vi "Average RGB Sub VI.vi"(5 "Coordinates of Overlay":cluster{"x-coord":i32, "y-coord":i32}, 7 "Transparency Factor":sgl, 8 "error in":errorcluster, 9 "Image":u32[][](array[numeric]), 10 "Overlay":u32[][](array[numeric]), 11 "Alpha Values (Transparency)":u8[][](array[numeric])) -> (0 "error out":errorcluster, 3 "Image Out":u32[][](array[numeric]))   [LabVIEW 2015]
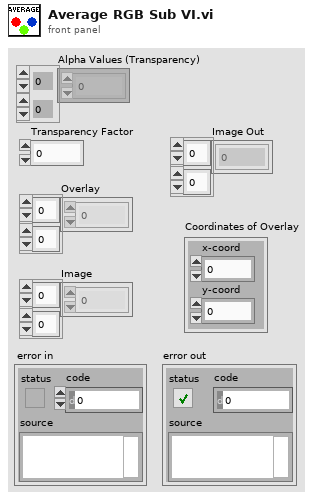
[diagram p1: front panel]
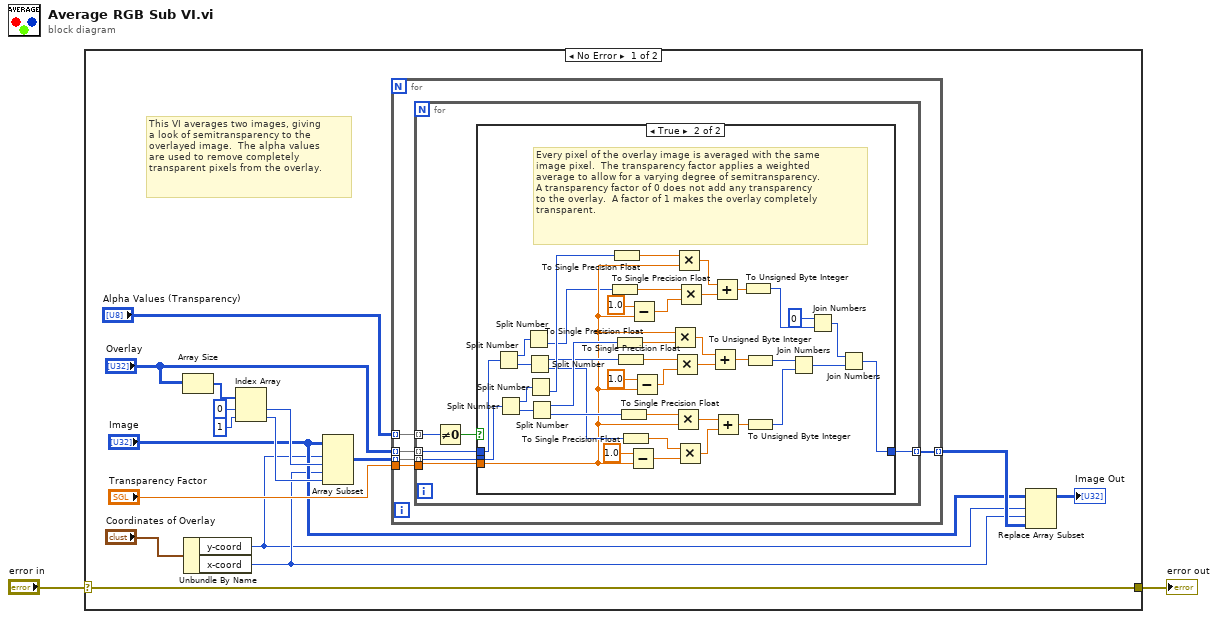
[diagram p0: block diagram]
diagram:
  n1 = case shown="No Error" "error in" {
    selector: "error in" -> [w6 w72]
    tunnel: [w6 w72] -> w1
    frame No Error {
      # "This VI averages two images, giving\na look of semitransparency to the\noverlayed image.  The alpha values \nare used to remove completely\ntransparent pixels from the overlay."
      n2 = Array Size(array="Overlay") -> (size(s)=w15:i32[])
      n3 = Unbundle By Name("Coordinates of Overlay") -> ("y-coord"=w7:i32, "x-coord"=w8:i32)
      n4 = Index Array(array=w15, index #1=0 ("index"), index #2=1 ("index")) -> (element #1=w13:i32, element #2=w14:i32)
      n5 = Array Subset(array="Image", index (row)=w7, length (row)=w13, index (col)=w8, length (col)=w14) -> (w9:u32[][])
      n6 = for {
        tunnel: w9 -> [w22] mode=indexing
        tunnel: "Overlay" -> [w23] mode=indexing
        tunnel: [w21] -> w12 mode=indexing
        tunnel: "Transparency Factor" -> [w20]
        tunnel: "Alpha Values (Transparency)" -> [w19] mode=indexing
        n7 = for {
          tunnel: w23 -> [w25] mode=indexing
          tunnel: w22 -> [w29] mode=indexing
          tunnel: [w28] -> w21 mode=indexing
          tunnel: w20 -> [w26]
          tunnel: w19 -> [w24] mode=indexing
          n8 = Not Equal To 0?(x=w24) -> (x != 0?=w27:bool)
          n9 = case shown="True" w27 {
            tunnel: w25 -> [_ w34]
            tunnel: w29 -> [w30 w35]
            tunnel: [w30 w37] -> w28
            tunnel: w26 -> [_ w36]
            frame False {
              # "Any pixel in the overaly image that has an alpha value\nof zero will not be averaged with the image.  This allows\nfor a completely transparent overlay pixel regardless of\nthe transparency factor.  This is especially useful when \na non-rectangular overlay template is used."
            }
            frame True {
              # "Every pixel of the overlay image is averaged with the same\nimage pixel.  The transparency factor applies a weighted\naverage to allow for a varying degree of semitransparency.\nA transparency factor of 0 does not add any transparency\nto the overlay.  A factor of 1 makes the overlay completely\ntransparent."
              n10 = Split Number(x=w34) -> (hi(x)=w33:u16, lo(x)=w31:u16)
              n11 = Split Number(x=w35) -> (hi(x)=w71:u16, lo(x)=w70:u16)
              n12 = Split Number(x=w33) -> (lo(x)=w32:u8)  [unwired: 1 out]
              n13 = Split Number(x=w31) -> (hi(x)=w43:u8, lo(x)=w39:u8)
              n14 = Split Number(x=w71) -> (lo(x)=w45:u8)  [unwired: 1 out]
              n15 = Split Number(x=w70) -> (hi(x)=w47:u8, lo(x)=w42:u8)
              n16 = To Single Precision Float(number=w32) -> (single precision float=w38:sgl)
              n17 = To Single Precision Float(number=w45) -> (single precision float=w48:sgl)
              n18 = To Single Precision Float(number=w47) -> (single precision float=w46:sgl)
              n19 = To Single Precision Float(number=w43) -> (single precision float=w44:sgl)
              n20 = To Single Precision Float(number=w42) -> (single precision float=w41:sgl)
              n21 = To Single Precision Float(number=w39) -> (single precision float=w40:sgl)
              n22 = Subtract(x=sgl 1.0, y=w36) -> (x-y=w61:sgl)
              n23 = Subtract(x=sgl 1.0 ("y"), y=w36) -> (x-y=w51:sgl)
              n24 = Subtract(x=sgl 1.0, y=w36) -> (x-y=w58:sgl)
              n25 = Multiply(x=w36, y=w46) -> (x*y=w56:sgl)
              n26 = Multiply(x=w44, y=w58) -> (x*y=w55:sgl)
              n27 = Multiply(x=w41, y=w36) -> (x*y=w62:sgl)
              n28 = Multiply(x=w48, y=w36) -> (x*y=w52:sgl)
              n29 = Multiply(x=w40, y=w61) -> (x*y=w63:sgl)
              n30 = Multiply(x=w38, y=w51) -> (x*y=w53:sgl)
              n31 = Add(x=w56, y=w55) -> (x+y=w57:sgl)
              n32 = Add(x=w52, y=w53) -> (x+y=w50:sgl)
              n33 = Add(x=w62, y=w63) -> (x+y=w59:sgl)
              n34 = To Unsigned Byte Integer(number=w50) -> (unsigned 8bit integer=w66:u8)
              n35 = To Unsigned Byte Integer(number=w57) -> (unsigned 8bit integer=w65:u8)
              n36 = To Unsigned Byte Integer(number=w59) -> (unsigned 8bit integer=w64:u8)
              n37 = Join Numbers(hi=w65, lo=w64) -> ((hi.lo)=w68:u16)
              n38 = Join Numbers(hi=u8 0, lo=w66) -> ((hi.lo)=w67:u16)
              n39 = Join Numbers(hi=w67, lo=w68) -> ((hi.lo)=w37:u32)
            }
          }
        }
      }
      n40 = Replace Array Subset(array="Image", new element=w12, index (row)=w7, index (col)=w8) -> (→"Image Out":u32[][])
    }
    frame Error {
    }
  }
  "error out" <- w1
